vi "Pulse Generator.vi"() -> ()   [LabVIEW 2012]
uses:
  <vilib>/DAQmx/read.llb/DAQmx Read (Digital Bool 1Line 1Point).vi
  <vilib>/Utility/file.llb/Write To Spreadsheet File (DBL).vi
  <vilib>/DAQmx/create/channels.llb/DAQmx Create Channel (DI-Digital Input).vi
  <vilib>/DAQmx/miscellaneous.llb/DAQmx Fill In Error Info.vi
panel:
  in  "Tab Control":T1(tab)
  in  "MW width Min":dbl=5e-08
  in  "MW width step size":dbl=2e-09
  in  "MW width Max":dbl=5e-07
  in  "Tau step size":dbl
  in  "Tau max":dbl
  in  "Tau min":dbl
  in  "Rabi Frequency":dbl
  in  "Rabi Frequency":dbl
  in  "Tau max":dbl
  in  "Tau min":dbl
  in  "Tau step size":dbl
  in  "Tau":dbl
  in  "Rabi Frequency  2":dbl
  in  "Tau' max 2":dbl
  in  "Tau' min 2":dbl
  in  "Tau' step size 2":dbl
  in  "AOM Rest time":dbl
  in  "Signal delay":dbl
  in  "N Loop":i32=25000
  in  "APD signal width":dbl
  out "Run":bool
  out "size(s)":i32=225
  in  "file path (dialog if empty)":path=path "C:/Users/Ouyang Group/Documents/Data/12-5-13/Rabi pulse sequence 7"
  in  "AOM Pulse length":dbl=3e-07
  in  "Path to spinapi.dll":path=path "C:/SpinCore/SpinAPI/dll/spinapi64.dll"
  in  "stop":bool
  in  "start/restart":bool
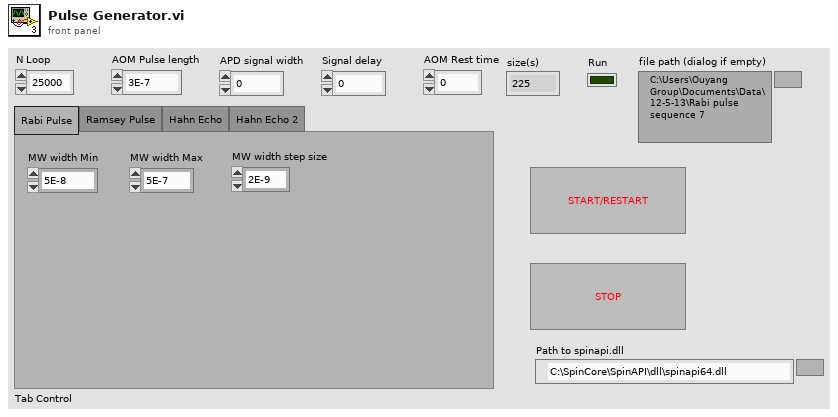
[diagram p1: front panel]
types:
  T1 = enum32{"Rabi Pulse", "Ramsey Pulse", "Hahn Echo", "Hahn Echo 2"}
  T2 = cluster{"Instruct Data":i32, "Op Code":i32, "Flags":bool[], "Comments":string, "Time (s)":dbl}[]
  T3 = cluster{"Instruct Data":i32, "Op Code":i32, "Flags":bool[], "Comments":string, "Time (s)":dbl}
  T4 = enum16{"Pulse Program", "Frequency Registers", "TX Phase Registers", "RX Phase Registers"}
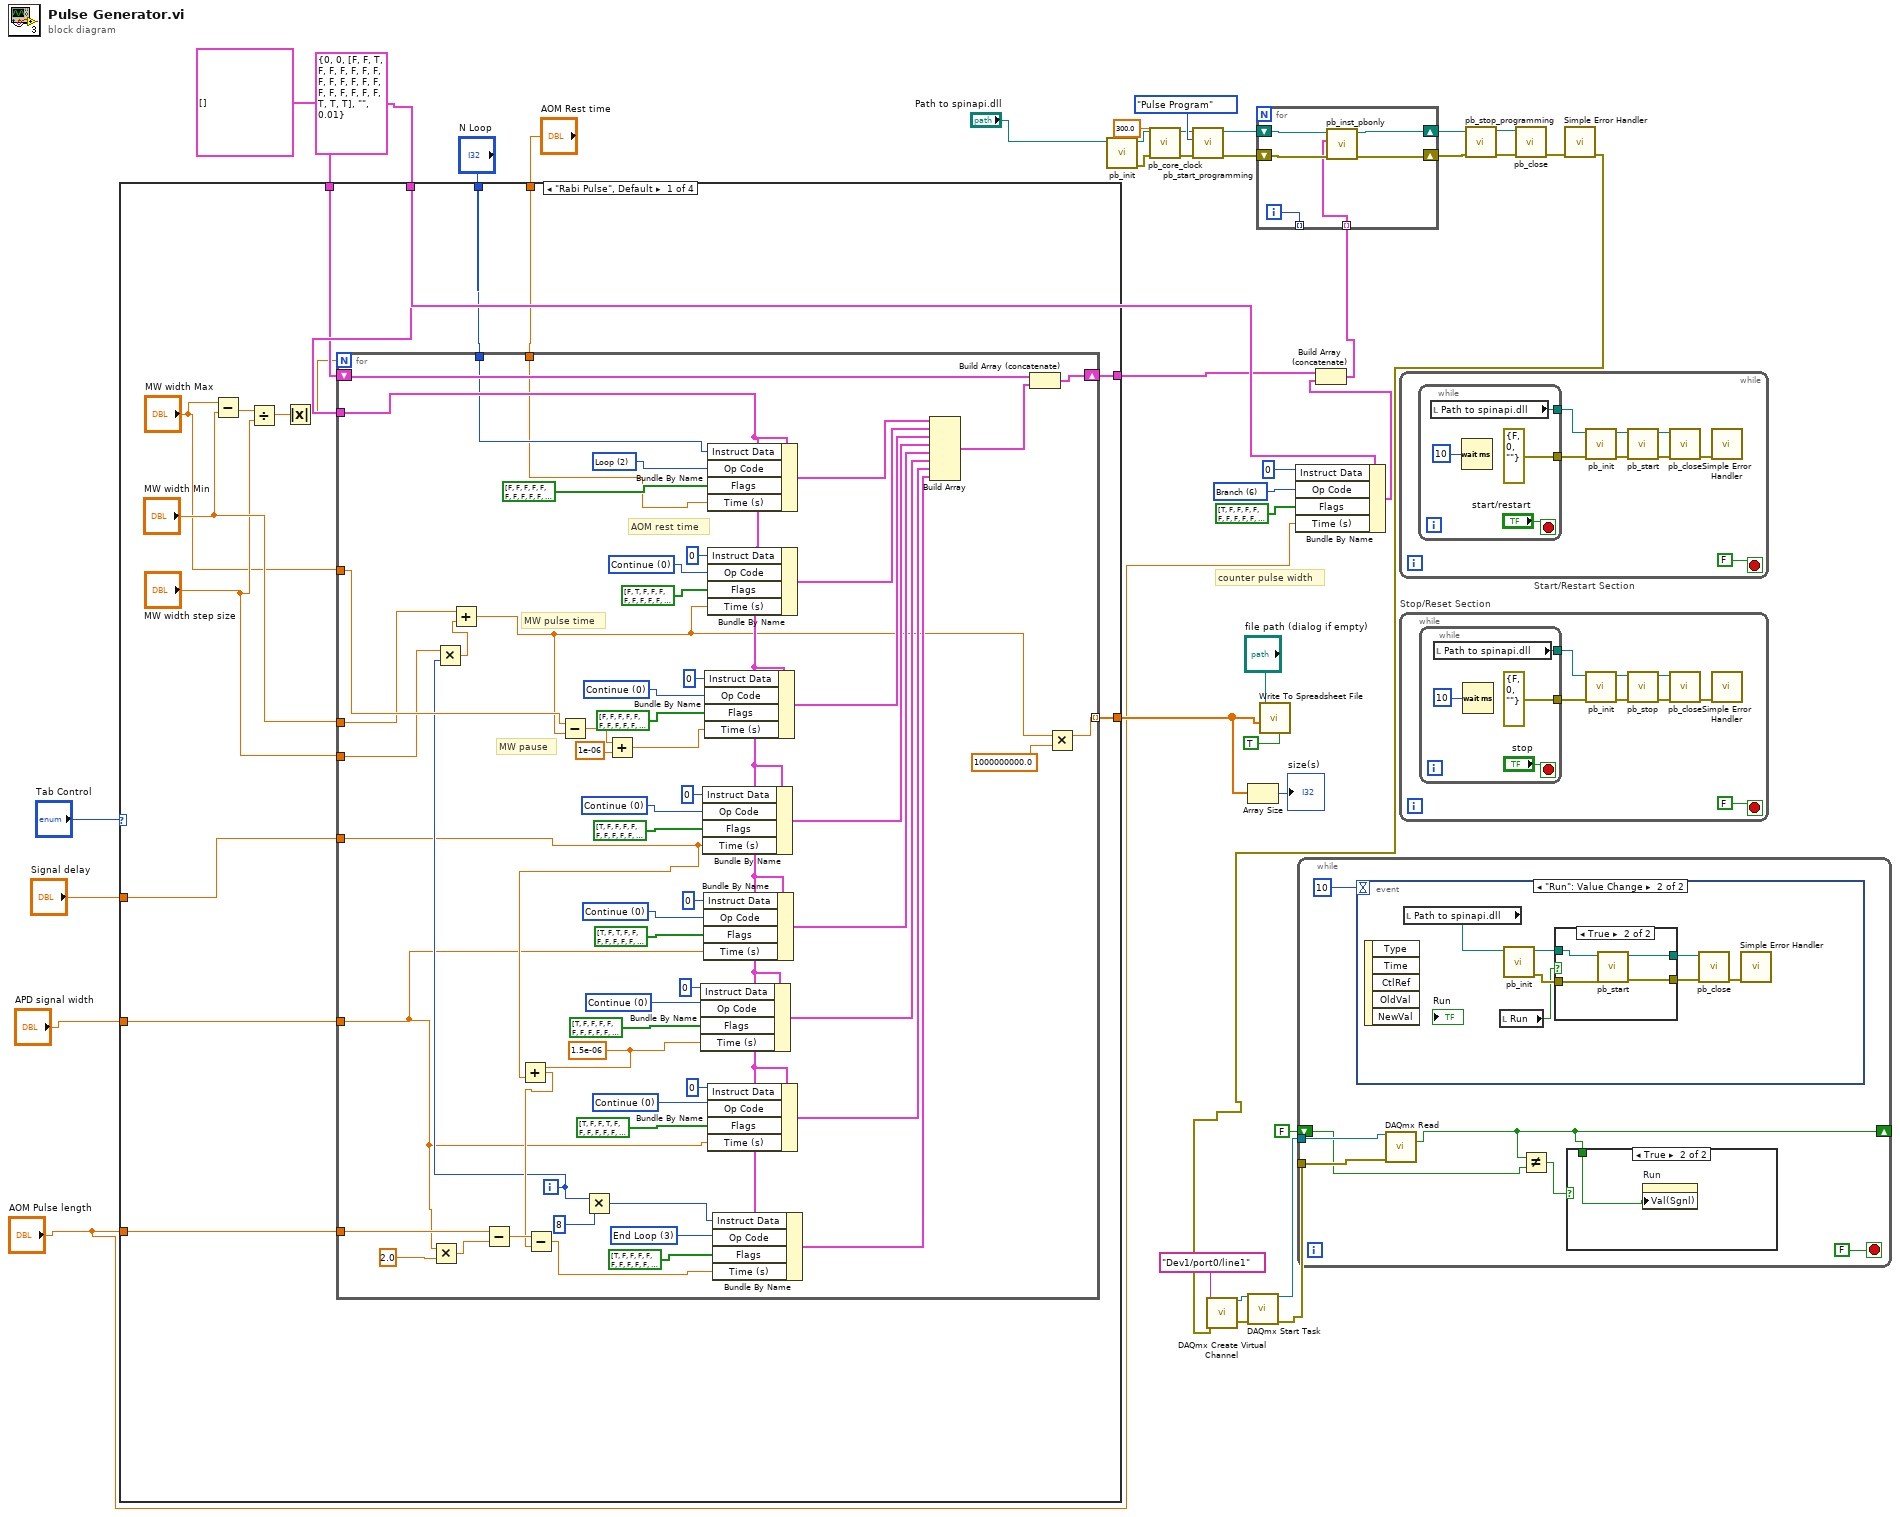
[diagram p0: block diagram]
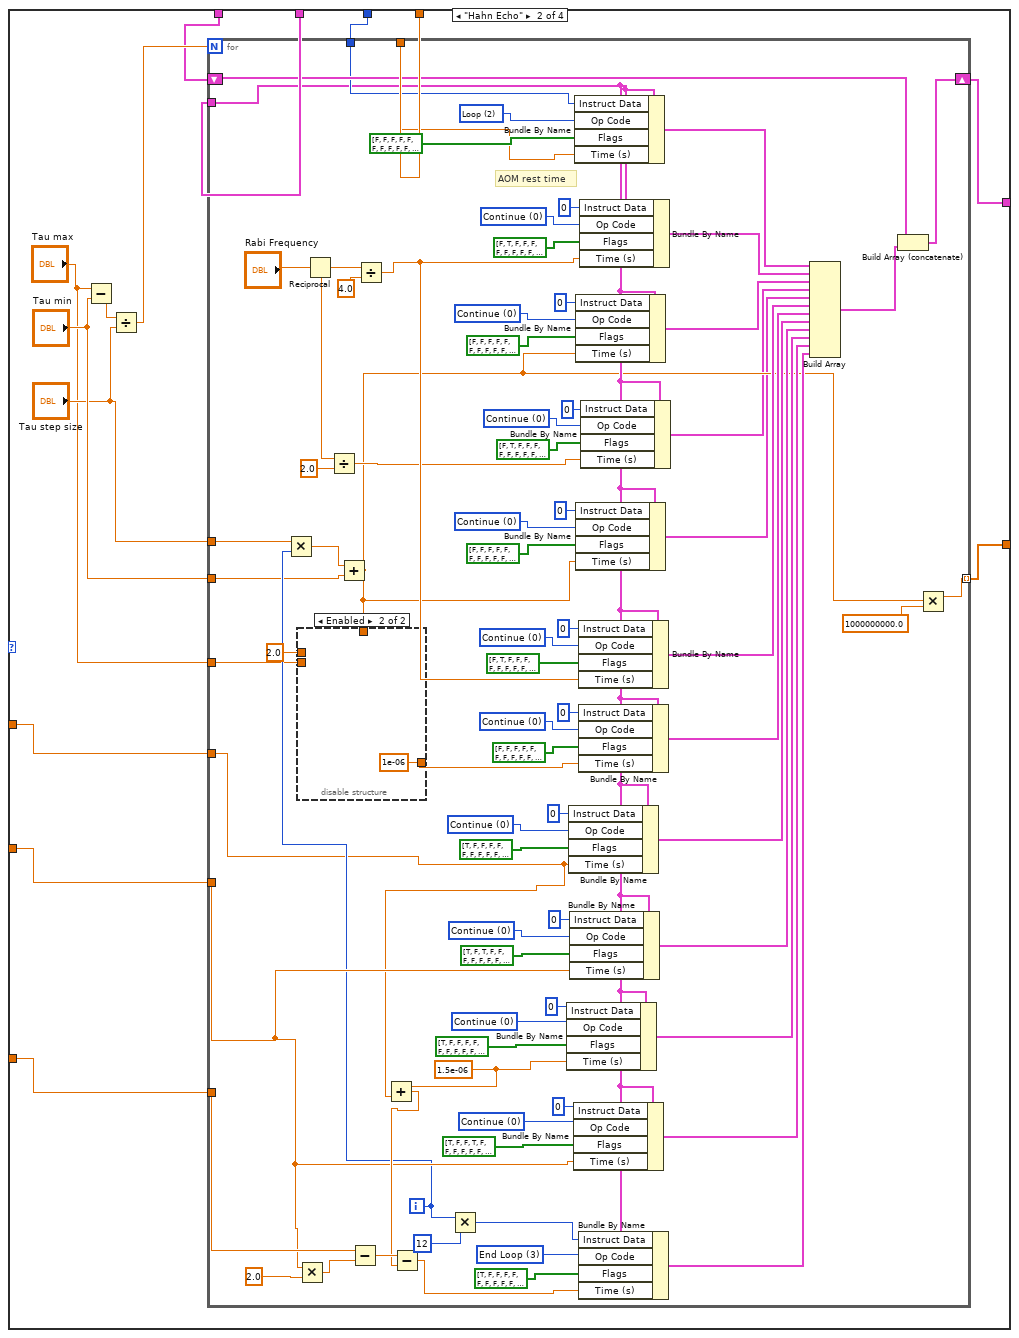
[diagram p2: hidden frame]
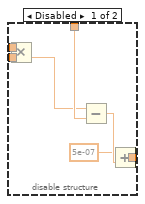
[diagram p3: hidden frame]
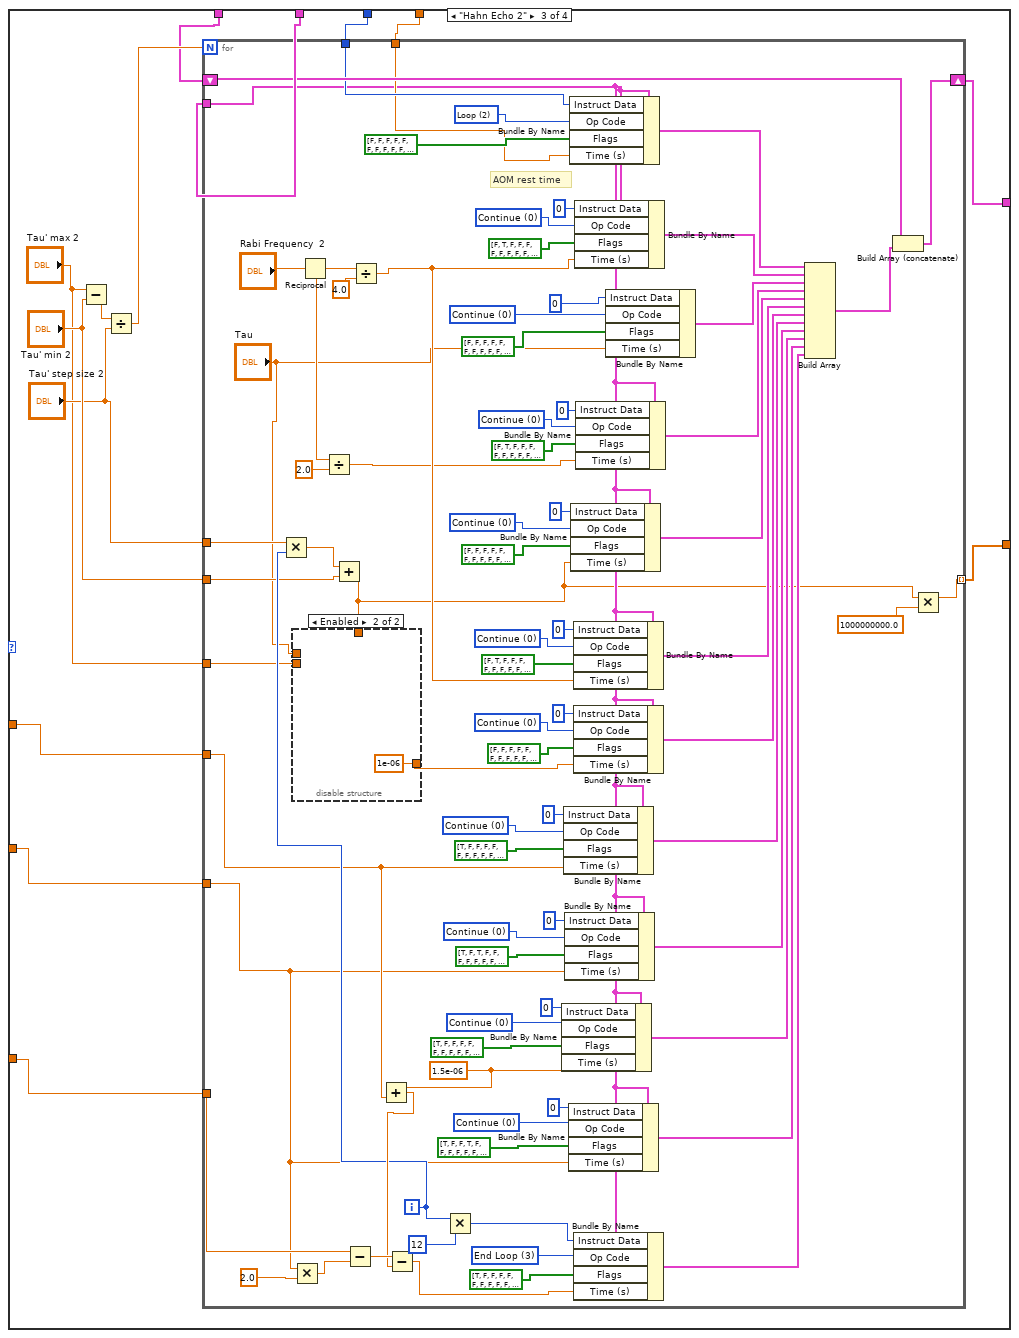
[diagram p4: hidden frame]
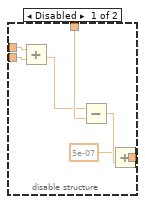
[diagram p5: hidden frame]
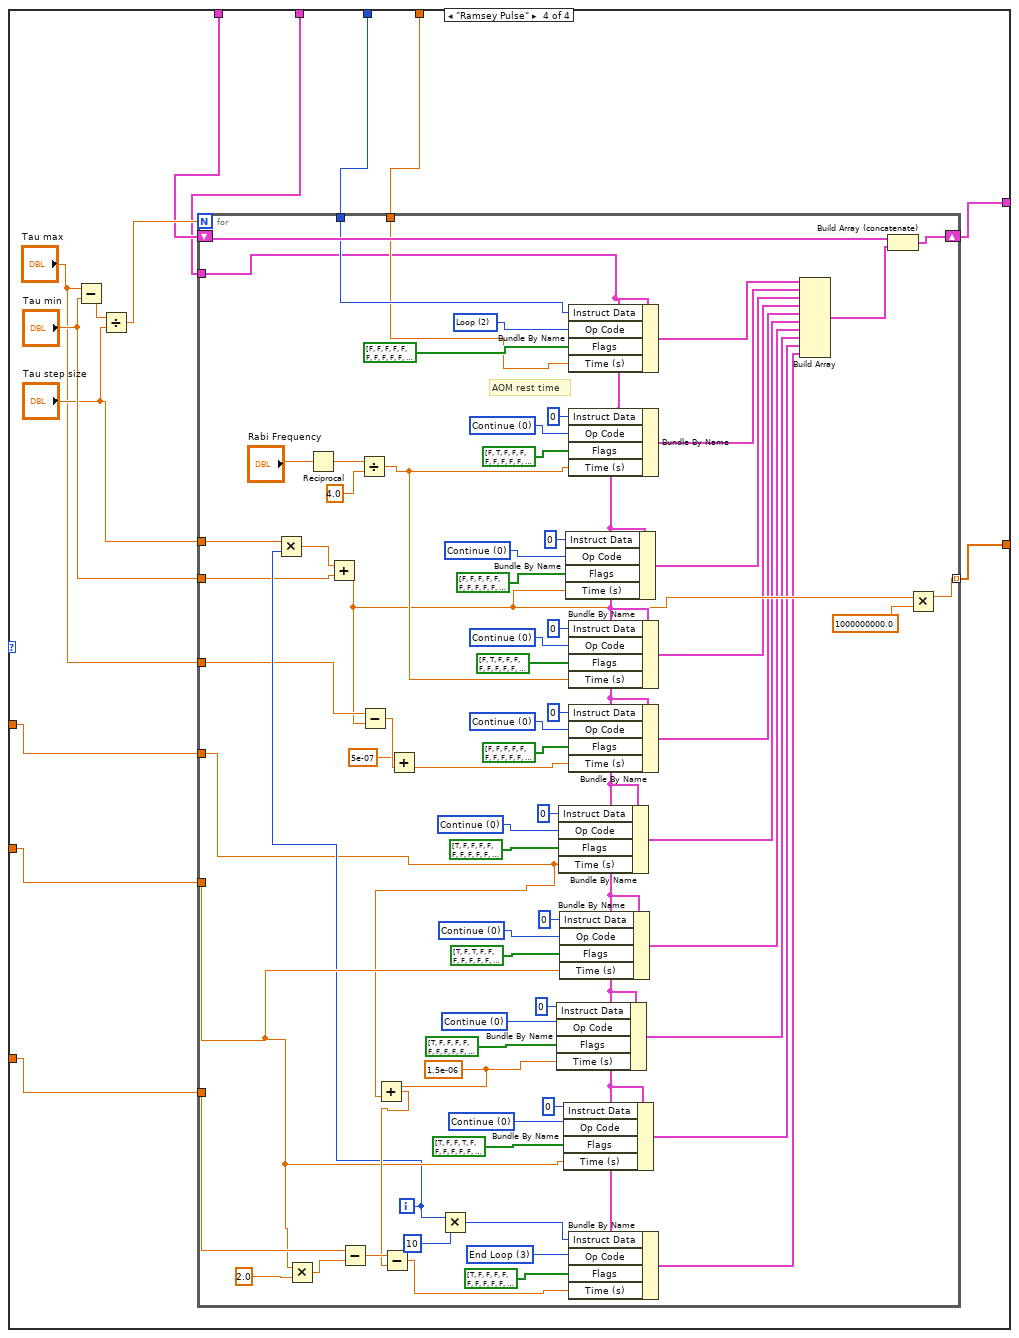
[diagram p6: hidden frame]
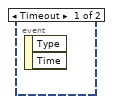
[diagram p7: hidden frame]
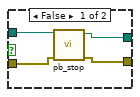
[diagram p8: hidden frame]
diagram:
  w13 = 6 items=["Continue", "Stop", "Loop", "End Loop", "JSR", "RTS", "Branch", "Long Delay", "Wait"] ("Op Code")
  w11 = T3 {"Instruct Data"=0, "Op Code"=0, "Flags"=[FALSE, FALSE, TRUE, FALSE, FALSE, FALSE, FALSE, FALSE, FALSE, FALSE, FALSE, FALSE, FALSE, FALSE, FALSE, FALSE, FALSE, FALSE, FALSE, FALSE, FALSE, TRUE, TRUE, TRUE], "Comments"="", "Time (s)"=0.01} ("PB Inst 2")
  # "counter pulse width"
  n1 = case shown="\"Rabi Pulse\", Default" "Tab Control" {
    tunnel: [w50 w115 w219 w328] -> w23
    tunnel: w11 -> [w48 w117 w222 w316]
    tunnel: [w47 w113 w220 w315] -> w9
    tunnel: T2 [] -> [w46 w118 w221 w317]
    tunnel: "N Loop" -> [w44 w116 w215 w327]
    tunnel: "AOM Rest time" -> [w43 w114 w214 w326]
    tunnel: "Signal delay" -> [w42 w121 w218 w323]
    tunnel: "AOM Pulse length" -> [w41 w119 w216 w325]
    tunnel: "APD signal width" -> [w40 w120 w217 w324]
    frame "Rabi Pulse", Default {
      n2 = Subtract(x="MW width Max", y="MW width Min") -> (x-y=w54:dbl)
      n3 = Divide(x=w54, y="MW width step size") -> (x/y=w53:dbl)
      n4 = Absolute Value(x=w53) -> (abs(x)=w45:dbl)
      n5 = for {
        N: w45 -> [_]
        tunnel: "MW width Min" -> [w61]
        tunnel: "MW width step size" -> [w62]
        tunnel: [w100] -> w50 mode=indexing
        tunnel: w48 -> [w81]
        shift-right: [w111] -> w47
        shift-left: w46 -> [w112]
        tunnel: "MW width Max" -> [w69]
        tunnel: w44 -> [w59]
        tunnel: w43 -> [w58]
        tunnel: w42 -> [w57]
        tunnel: w41 -> [w56]
        tunnel: w40 -> [w55]
        i -> [w63]
        w71 = 0 items=["Continue", "Stop", "Loop", "End Loop", "JSR", "RTS", "Branch", "Long Delay", "Wait"] ("Op Code")
        w74 = 2 items=["Continue", "Stop", "Loop", "End Loop", "JSR", "RTS", "Branch", "Long Delay", "Wait"] ("Op Code")
        w83 = 0 items=["Continue", "Stop", "Loop", "End Loop", "JSR", "RTS", "Branch", "Long Delay", "Wait"] ("Op Code")
        w86 = 1.5e-06 ("Time (s)")
        w90 = 0 items=["Continue", "Stop", "Loop", "End Loop", "JSR", "RTS", "Branch", "Long Delay", "Wait"] ("Op Code")
        w95 = 3 items=["Continue", "Stop", "Loop", "End Loop", "JSR", "RTS", "Branch", "Long Delay", "Wait"] ("Op Code")
        w98 = 0 items=["Continue", "Stop", "Loop", "End Loop", "JSR", "RTS", "Branch", "Long Delay", "Wait"] ("Op Code")
        w106 = 0 items=["Continue", "Stop", "Loop", "End Loop", "JSR", "RTS", "Branch", "Long Delay", "Wait"] ("Op Code")
        w109 = 0 items=["Continue", "Stop", "Loop", "End Loop", "JSR", "RTS", "Branch", "Long Delay", "Wait"] ("Op Code")
        # "MW pause"
        # "AOM rest time"
        # "MW pulse time"
        n6 = Multiply(x=w55, y=2.0) -> (x*y=w91:dbl)
        n7 = Multiply(x=w62, y=w63) -> (x*y=w64:dbl)
        n8 = Add(x=w61, y=w64) -> (x+y=w60:dbl)
        n9 = Subtract(x=w56, y=w91) -> (x-y=w87:dbl)
        n10 = Add(x=w86, y=w57) -> (x+y=w75:dbl)
        n11 = Subtract(x=w87, y=w75) -> (x-y=w85:dbl)
        n12 = Subtract(x=w69, y=w60) -> (x-y=w68:dbl)
        n13 = Multiply(x=w63, y=8) -> (x*y=w65:i32)
        n14 = Add(x=w68, y=1e-06) -> (x+y=w66:dbl)
        n15 = Bundle By Name(cluster=w81, "Instruct Data"=0, "Op Code"=w98, "Flags"=bool[] [TRUE, FALSE, FALSE, FALSE, FALSE, FALSE, FALSE, FALSE, FALSE, FALSE, FALSE, FALSE, FALSE, FALSE, FALSE, FALSE, FALSE, FALSE, FALSE, FALSE, FALSE, TRUE, TRUE, TRUE], "Time (s)"=w86) -> (w76:T3)
        n16 = Bundle By Name(cluster=w81, "Instruct Data"=0, "Op Code"=w83, "Flags"=bool[] [TRUE, FALSE, FALSE, FALSE, FALSE, FALSE, FALSE, FALSE, FALSE, FALSE, FALSE, FALSE, FALSE, FALSE, FALSE, FALSE, FALSE, FALSE, FALSE, FALSE, FALSE, TRUE, TRUE, TRUE], "Time (s)"=w57) -> (w79:T3)
        n17 = Bundle By Name(cluster=w81, "Instruct Data"=0, "Op Code"=w106, "Flags"=bool[] [TRUE, FALSE, TRUE, FALSE, FALSE, FALSE, FALSE, FALSE, FALSE, FALSE, FALSE, FALSE, FALSE, FALSE, FALSE, FALSE, FALSE, FALSE, FALSE, FALSE, FALSE, TRUE, TRUE, TRUE], "Time (s)"=w55) -> (w80:T3)
        n18 = Bundle By Name(cluster=w81, "Instruct Data"=0, "Op Code"=w109, "Flags"=bool[] [FALSE, FALSE, FALSE, FALSE, FALSE, FALSE, FALSE, FALSE, FALSE, FALSE, FALSE, FALSE, FALSE, FALSE, FALSE, FALSE, FALSE, FALSE, FALSE, FALSE, FALSE, TRUE, TRUE, TRUE], "Time (s)"=w66) -> (w103:T3)
        n19 = Bundle By Name(cluster=w81, "Instruct Data"=w59, "Op Code"=w74, "Flags"=bool[] [FALSE, FALSE, FALSE, FALSE, FALSE, FALSE, FALSE, FALSE, FALSE, FALSE, FALSE, FALSE, FALSE, FALSE, FALSE, FALSE, FALSE, FALSE, FALSE, FALSE, FALSE, TRUE, TRUE, TRUE], "Time (s)"=w58) -> (w105:T3)
        n20 = Bundle By Name(cluster=w81, "Instruct Data"=0, "Op Code"=w71, "Flags"=bool[] [FALSE, TRUE, FALSE, FALSE, FALSE, FALSE, FALSE, FALSE, FALSE, FALSE, FALSE, FALSE, FALSE, FALSE, FALSE, FALSE, FALSE, FALSE, FALSE, FALSE, FALSE, TRUE, TRUE, TRUE], "Time (s)"=w60) -> (w104:T3)
        n21 = Bundle By Name(cluster=w81, "Instruct Data"=0, "Op Code"=w90, "Flags"=bool[] [TRUE, FALSE, FALSE, TRUE, FALSE, FALSE, FALSE, FALSE, FALSE, FALSE, FALSE, FALSE, FALSE, FALSE, FALSE, FALSE, FALSE, FALSE, FALSE, FALSE, FALSE, TRUE, TRUE, TRUE], "Time (s)"=w55) -> (w77:T3)
        n22 = Bundle By Name(cluster=w81, "Instruct Data"=w65, "Op Code"=w95, "Flags"=bool[] [TRUE, FALSE, FALSE, FALSE, FALSE, FALSE, FALSE, FALSE, FALSE, FALSE, FALSE, FALSE, FALSE, FALSE, FALSE, FALSE, FALSE, FALSE, FALSE, FALSE, FALSE, TRUE, TRUE, TRUE], "Time (s)"=w85) -> (w78:T3)
        n23 = Build Array(w105, w104, w103, w79, w80, w76, w77, w78) -> (w101:T2)
        n24 = Build Array (concatenate)(w112, w101) -> (w111:T2)
        n25 = Multiply(x=w60, y=1000000000.0) -> (x*y=w100:dbl)
      }
    }
    frame "Hahn Echo" {
      n26 = Subtract(x="Tau max", y="Tau min") -> (x-y=w126:dbl)
      n27 = Divide(x=w126, y="Tau step size") -> (x/y=w125:dbl)
      n28 = for {
        N: w125 -> [_]
        tunnel: [w197] -> w115 mode=indexing
        tunnel: w117 -> [w134]
        shift-right: [w146] -> w113
        shift-left: w118 -> [w205]
        tunnel: w116 -> [w171]
        tunnel: w114 -> [w170]
        tunnel: w121 -> [w145]
        tunnel: w119 -> [w169]
        tunnel: w120 -> [w168]
        tunnel: "Tau min" -> [w165]
        tunnel: "Tau step size" -> [w167]
        tunnel: "Tau max" -> [w154]
        i -> [w166]
        w136 = 0 items=["Continue", "Stop", "Loop", "End Loop", "JSR", "RTS", "Branch", "Long Delay", "Wait"] ("Op Code")
        w142 = 0 items=["Continue", "Stop", "Loop", "End Loop", "JSR", "RTS", "Branch", "Long Delay", "Wait"] ("Op Code")
        w156 = 0 items=["Continue", "Stop", "Loop", "End Loop", "JSR", "RTS", "Branch", "Long Delay", "Wait"] ("Op Code")
        w160 = 0 items=["Continue", "Stop", "Loop", "End Loop", "JSR", "RTS", "Branch", "Long Delay", "Wait"] ("Op Code")
        w174 = 0 items=["Continue", "Stop", "Loop", "End Loop", "JSR", "RTS", "Branch", "Long Delay", "Wait"] ("Op Code")
        w177 = 2 items=["Continue", "Stop", "Loop", "End Loop", "JSR", "RTS", "Branch", "Long Delay", "Wait"] ("Op Code")
        w180 = 0 items=["Continue", "Stop", "Loop", "End Loop", "JSR", "RTS", "Branch", "Long Delay", "Wait"] ("Op Code")
        w183 = 1.5e-06 ("Time (s)")
        w187 = 0 items=["Continue", "Stop", "Loop", "End Loop", "JSR", "RTS", "Branch", "Long Delay", "Wait"] ("Op Code")
        w192 = 3 items=["Continue", "Stop", "Loop", "End Loop", "JSR", "RTS", "Branch", "Long Delay", "Wait"] ("Op Code")
        w195 = 0 items=["Continue", "Stop", "Loop", "End Loop", "JSR", "RTS", "Branch", "Long Delay", "Wait"] ("Op Code")
        w200 = 0 items=["Continue", "Stop", "Loop", "End Loop", "JSR", "RTS", "Branch", "Long Delay", "Wait"] ("Op Code")
        w203 = 0 items=["Continue", "Stop", "Loop", "End Loop", "JSR", "RTS", "Branch", "Long Delay", "Wait"] ("Op Code")
        # "AOM rest time"
        n29 = Multiply(x=w167, y=w166) -> (x*y=w164:dbl)
        n30 = Multiply(x=w168, y=2.0) -> (x*y=w188:dbl)
        n31 = Reciprocal(x="Rabi Frequency") -> (1/x=w140:dbl)
        n32 = Divide(x=w140, y=2.0) -> (x/y=w138:dbl)
        n33 = Add(x=w164, y=w165) -> (x+y=w133:dbl)
        n34 = disable-structure shown="Enabled" {
          disable-tunnel: w154 -> [w212 _]
          disable-tunnel: [w210 1e-06] -> w144
          disable-tunnel: w133 -> [w208 _]
          disable-tunnel: 2.0 ("x") -> [w206 _]
          frame Disabled {
            n35 = Multiply(x=w206, y=w212) -> (x*y=w207:dbl)
            n36 = Subtract(x=w207, y=w208) -> (x-y=w211:dbl)
            n37 = Add(x=5e-07, y=w211) -> (x+y=w210:dbl)
          }
          frame Enabled {
          }
        }
        n38 = Subtract(x=w169, y=w188) -> (x-y=w184:dbl)
        n39 = Divide(x=w140, y=4.0) -> (x/y=w158:dbl)
        n40 = Add(x=w183, y=w145) -> (x+y=w178:dbl)
        n41 = Subtract(x=w184, y=w178) -> (x-y=w182:dbl)
        n42 = Multiply(x=w166, y=12) -> (x*y=w172:i32)
        n43 = Bundle By Name(cluster=w134, "Instruct Data"=0, "Op Code"=w195, "Flags"=bool[] [TRUE, FALSE, FALSE, FALSE, FALSE, FALSE, FALSE, FALSE, FALSE, FALSE, FALSE, FALSE, FALSE, FALSE, FALSE, FALSE, FALSE, FALSE, FALSE, FALSE, FALSE, TRUE, TRUE, TRUE], "Time (s)"=w183) -> (w149:T3)
        n44 = Bundle By Name(cluster=w134, "Instruct Data"=0, "Op Code"=w180, "Flags"=bool[] [TRUE, FALSE, FALSE, FALSE, FALSE, FALSE, FALSE, FALSE, FALSE, FALSE, FALSE, FALSE, FALSE, FALSE, FALSE, FALSE, FALSE, FALSE, FALSE, FALSE, FALSE, TRUE, TRUE, TRUE], "Time (s)"=w145) -> (w151:T3)
        n45 = Bundle By Name(cluster=w134, "Instruct Data"=0, "Op Code"=w200, "Flags"=bool[] [TRUE, FALSE, TRUE, FALSE, FALSE, FALSE, FALSE, FALSE, FALSE, FALSE, FALSE, FALSE, FALSE, FALSE, FALSE, FALSE, FALSE, FALSE, FALSE, FALSE, FALSE, TRUE, TRUE, TRUE], "Time (s)"=w168) -> (w150:T3)
        n46 = Bundle By Name(cluster=w134, "Instruct Data"=0, "Op Code"=w187, "Flags"=bool[] [TRUE, FALSE, FALSE, TRUE, FALSE, FALSE, FALSE, FALSE, FALSE, FALSE, FALSE, FALSE, FALSE, FALSE, FALSE, FALSE, FALSE, FALSE, FALSE, FALSE, FALSE, TRUE, TRUE, TRUE], "Time (s)"=w168) -> (w148:T3)
        n47 = Bundle By Name(cluster=w134, "Instruct Data"=w171, "Op Code"=w177, "Flags"=bool[] [FALSE, FALSE, FALSE, FALSE, FALSE, FALSE, FALSE, FALSE, FALSE, FALSE, FALSE, FALSE, FALSE, FALSE, FALSE, FALSE, FALSE, FALSE, FALSE, FALSE, FALSE, TRUE, TRUE, TRUE], "Time (s)"=w170) -> (w127:T3)
        n48 = Bundle By Name(cluster=w134, "Instruct Data"=0, "Op Code"=w203, "Flags"=bool[] [FALSE, FALSE, FALSE, FALSE, FALSE, FALSE, FALSE, FALSE, FALSE, FALSE, FALSE, FALSE, FALSE, FALSE, FALSE, FALSE, FALSE, FALSE, FALSE, FALSE, FALSE, TRUE, TRUE, TRUE], "Time (s)"=w133) -> (w129:T3)
        n49 = Bundle By Name(cluster=w134, "Instruct Data"=0, "Op Code"=w136, "Flags"=bool[] [FALSE, FALSE, FALSE, FALSE, FALSE, FALSE, FALSE, FALSE, FALSE, FALSE, FALSE, FALSE, FALSE, FALSE, FALSE, FALSE, FALSE, FALSE, FALSE, FALSE, FALSE, TRUE, TRUE, TRUE], "Time (s)"=w133) -> (w131:T3)
        n50 = Bundle By Name(cluster=w134, "Instruct Data"=0, "Op Code"=w160, "Flags"=bool[] [FALSE, TRUE, FALSE, FALSE, FALSE, FALSE, FALSE, FALSE, FALSE, FALSE, FALSE, FALSE, FALSE, FALSE, FALSE, FALSE, FALSE, FALSE, FALSE, FALSE, FALSE, TRUE, TRUE, TRUE], "Time (s)"=w158) -> (w153:T3)
        n51 = Bundle By Name(cluster=w134, "Instruct Data"=0, "Op Code"=w156, "Flags"=bool[] [FALSE, FALSE, FALSE, FALSE, FALSE, FALSE, FALSE, FALSE, FALSE, FALSE, FALSE, FALSE, FALSE, FALSE, FALSE, FALSE, FALSE, FALSE, FALSE, FALSE, FALSE, TRUE, TRUE, TRUE], "Time (s)"=w144) -> (w152:T3)
        n52 = Bundle By Name(cluster=w134, "Instruct Data"=w172, "Op Code"=w192, "Flags"=bool[] [TRUE, FALSE, FALSE, FALSE, FALSE, FALSE, FALSE, FALSE, FALSE, FALSE, FALSE, FALSE, FALSE, FALSE, FALSE, FALSE, FALSE, FALSE, FALSE, FALSE, FALSE, TRUE, TRUE, TRUE], "Time (s)"=w182) -> (w147:T3)
        n53 = Bundle By Name(cluster=w134, "Instruct Data"=0, "Op Code"=w174, "Flags"=bool[] [FALSE, TRUE, FALSE, FALSE, FALSE, FALSE, FALSE, FALSE, FALSE, FALSE, FALSE, FALSE, FALSE, FALSE, FALSE, FALSE, FALSE, FALSE, FALSE, FALSE, FALSE, TRUE, TRUE, TRUE], "Time (s)"=w158) -> (w128:T3)
        n54 = Bundle By Name(cluster=w134, "Instruct Data"=0, "Op Code"=w142, "Flags"=bool[] [FALSE, TRUE, FALSE, FALSE, FALSE, FALSE, FALSE, FALSE, FALSE, FALSE, FALSE, FALSE, FALSE, FALSE, FALSE, FALSE, FALSE, FALSE, FALSE, FALSE, FALSE, TRUE, TRUE, TRUE], "Time (s)"=w138) -> (w130:T3)
        n55 = Build Array(w127, w128, w129, w130, w131, w153, w152, w151, w150, w149, w148, w147) -> (w198:T2)
        n56 = Build Array (concatenate)(w205, w198) -> (w146:T2)
        n57 = Multiply(x=w133, y=1000000000.0) -> (x*y=w197:dbl)
      }
    }
    frame "Hahn Echo 2" {
      n58 = Subtract(x="Tau' max 2", y="Tau' min 2") -> (x-y=w227:dbl)
      n59 = Divide(x=w227, y="Tau' step size 2") -> (x/y=w226:dbl)
      n60 = for {
        N: w226 -> [_]
        tunnel: [w298] -> w219 mode=indexing
        tunnel: w222 -> [w236]
        shift-right: [w248] -> w220
        shift-left: w221 -> [w306]
        tunnel: w215 -> [w272]
        tunnel: w214 -> [w271]
        tunnel: w218 -> [w247]
        tunnel: w216 -> [w270]
        tunnel: w217 -> [w228]
        tunnel: "Tau' min 2" -> [w267]
        tunnel: "Tau' step size 2" -> [w269]
        tunnel: "Tau' max 2" -> [w256]
        i -> [w268]
        w238 = 0 items=["Continue", "Stop", "Loop", "End Loop", "JSR", "RTS", "Branch", "Long Delay", "Wait"] ("Op Code")
        w244 = 0 items=["Continue", "Stop", "Loop", "End Loop", "JSR", "RTS", "Branch", "Long Delay", "Wait"] ("Op Code")
        w258 = 0 items=["Continue", "Stop", "Loop", "End Loop", "JSR", "RTS", "Branch", "Long Delay", "Wait"] ("Op Code")
        w262 = 0 items=["Continue", "Stop", "Loop", "End Loop", "JSR", "RTS", "Branch", "Long Delay", "Wait"] ("Op Code")
        w275 = 0 items=["Continue", "Stop", "Loop", "End Loop", "JSR", "RTS", "Branch", "Long Delay", "Wait"] ("Op Code")
        w278 = 2 items=["Continue", "Stop", "Loop", "End Loop", "JSR", "RTS", "Branch", "Long Delay", "Wait"] ("Op Code")
        w281 = 0 items=["Continue", "Stop", "Loop", "End Loop", "JSR", "RTS", "Branch", "Long Delay", "Wait"] ("Op Code")
        w284 = 1.5e-06 ("Time (s)")
        w288 = 0 items=["Continue", "Stop", "Loop", "End Loop", "JSR", "RTS", "Branch", "Long Delay", "Wait"] ("Op Code")
        w293 = 3 items=["Continue", "Stop", "Loop", "End Loop", "JSR", "RTS", "Branch", "Long Delay", "Wait"] ("Op Code")
        w296 = 0 items=["Continue", "Stop", "Loop", "End Loop", "JSR", "RTS", "Branch", "Long Delay", "Wait"] ("Op Code")
        w301 = 0 items=["Continue", "Stop", "Loop", "End Loop", "JSR", "RTS", "Branch", "Long Delay", "Wait"] ("Op Code")
        w304 = 0 items=["Continue", "Stop", "Loop", "End Loop", "JSR", "RTS", "Branch", "Long Delay", "Wait"] ("Op Code")
        # "AOM rest time"
        n61 = Multiply(x=w269, y=w268) -> (x*y=w266:dbl)
        n62 = Multiply(x=w228, y=2.0) -> (x*y=w289:dbl)
        n63 = Reciprocal(x="Rabi Frequency  2") -> (1/x=w242:dbl)
        n64 = Divide(x=w242, y=2.0) -> (x/y=w240:dbl)
        n65 = Add(x=w266, y=w267) -> (x+y=w230:dbl)
        n66 = disable-structure shown="Enabled" {
          disable-tunnel: w256 -> [w313 _]
          disable-tunnel: [w311 1e-06] -> w246
          disable-tunnel: w230 -> [w309 _]
          disable-tunnel: "Tau" -> [w307 _]
          frame Disabled {
            n67 = Add(x=w307, y=w313) -> (x+y=w308:dbl)
            n68 = Subtract(x=w308, y=w309) -> (x-y=w312:dbl)
            n69 = Add(x=5e-07, y=w312) -> (x+y=w311:dbl)
          }
          frame Enabled {
          }
        }
        n70 = Subtract(x=w270, y=w289) -> (x-y=w285:dbl)
        n71 = Divide(x=w242, y=4.0) -> (x/y=w260:dbl)
        n72 = Add(x=w284, y=w247) -> (x+y=w279:dbl)
        n73 = Subtract(x=w285, y=w279) -> (x-y=w283:dbl)
        n74 = Multiply(x=w268, y=12) -> (x*y=w273:i32)
        n75 = Bundle By Name(cluster=w236, "Instruct Data"=0, "Op Code"=w296, "Flags"=bool[] [TRUE, FALSE, FALSE, FALSE, FALSE, FALSE, FALSE, FALSE, FALSE, FALSE, FALSE, FALSE, FALSE, FALSE, FALSE, FALSE, FALSE, FALSE, FALSE, FALSE, FALSE, TRUE, TRUE, TRUE], "Time (s)"=w284) -> (w251:T3)
        n76 = Bundle By Name(cluster=w236, "Instruct Data"=0, "Op Code"=w281, "Flags"=bool[] [TRUE, FALSE, FALSE, FALSE, FALSE, FALSE, FALSE, FALSE, FALSE, FALSE, FALSE, FALSE, FALSE, FALSE, FALSE, FALSE, FALSE, FALSE, FALSE, FALSE, FALSE, TRUE, TRUE, TRUE], "Time (s)"=w247) -> (w253:T3)
        n77 = Bundle By Name(cluster=w236, "Instruct Data"=0, "Op Code"=w301, "Flags"=bool[] [TRUE, FALSE, TRUE, FALSE, FALSE, FALSE, FALSE, FALSE, FALSE, FALSE, FALSE, FALSE, FALSE, FALSE, FALSE, FALSE, FALSE, FALSE, FALSE, FALSE, FALSE, TRUE, TRUE, TRUE], "Time (s)"=w228) -> (w252:T3)
        n78 = Bundle By Name(cluster=w236, "Instruct Data"=0, "Op Code"=w288, "Flags"=bool[] [TRUE, FALSE, FALSE, TRUE, FALSE, FALSE, FALSE, FALSE, FALSE, FALSE, FALSE, FALSE, FALSE, FALSE, FALSE, FALSE, FALSE, FALSE, FALSE, FALSE, FALSE, TRUE, TRUE, TRUE], "Time (s)"=w228) -> (w250:T3)
        n79 = Bundle By Name(cluster=w236, "Instruct Data"=w272, "Op Code"=w278, "Flags"=bool[] [FALSE, FALSE, FALSE, FALSE, FALSE, FALSE, FALSE, FALSE, FALSE, FALSE, FALSE, FALSE, FALSE, FALSE, FALSE, FALSE, FALSE, FALSE, FALSE, FALSE, FALSE, TRUE, TRUE, TRUE], "Time (s)"=w271) -> (w231:T3)
        n80 = Bundle By Name(cluster=w236, "Instruct Data"=0, "Op Code"=w238, "Flags"=bool[] [FALSE, FALSE, FALSE, FALSE, FALSE, FALSE, FALSE, FALSE, FALSE, FALSE, FALSE, FALSE, FALSE, FALSE, FALSE, FALSE, FALSE, FALSE, FALSE, FALSE, FALSE, TRUE, TRUE, TRUE], "Time (s)"=w230) -> (w235:T3)
        n81 = Bundle By Name(cluster=w236, "Instruct Data"=0, "Op Code"=w262, "Flags"=bool[] [FALSE, TRUE, FALSE, FALSE, FALSE, FALSE, FALSE, FALSE, FALSE, FALSE, FALSE, FALSE, FALSE, FALSE, FALSE, FALSE, FALSE, FALSE, FALSE, FALSE, FALSE, TRUE, TRUE, TRUE], "Time (s)"=w260) -> (w255:T3)
        n82 = Bundle By Name(cluster=w236, "Instruct Data"=0, "Op Code"=w258, "Flags"=bool[] [FALSE, FALSE, FALSE, FALSE, FALSE, FALSE, FALSE, FALSE, FALSE, FALSE, FALSE, FALSE, FALSE, FALSE, FALSE, FALSE, FALSE, FALSE, FALSE, FALSE, FALSE, TRUE, TRUE, TRUE], "Time (s)"=w246) -> (w254:T3)
        n83 = Bundle By Name(cluster=w236, "Instruct Data"=w273, "Op Code"=w293, "Flags"=bool[] [TRUE, FALSE, FALSE, FALSE, FALSE, FALSE, FALSE, FALSE, FALSE, FALSE, FALSE, FALSE, FALSE, FALSE, FALSE, FALSE, FALSE, FALSE, FALSE, FALSE, FALSE, TRUE, TRUE, TRUE], "Time (s)"=w283) -> (w249:T3)
        n84 = Bundle By Name(cluster=w236, "Instruct Data"=0, "Op Code"=w275, "Flags"=bool[] [FALSE, TRUE, FALSE, FALSE, FALSE, FALSE, FALSE, FALSE, FALSE, FALSE, FALSE, FALSE, FALSE, FALSE, FALSE, FALSE, FALSE, FALSE, FALSE, FALSE, FALSE, TRUE, TRUE, TRUE], "Time (s)"=w260) -> (w232:T3)
        n85 = Bundle By Name(cluster=w236, "Instruct Data"=0, "Op Code"=w244, "Flags"=bool[] [FALSE, TRUE, FALSE, FALSE, FALSE, FALSE, FALSE, FALSE, FALSE, FALSE, FALSE, FALSE, FALSE, FALSE, FALSE, FALSE, FALSE, FALSE, FALSE, FALSE, FALSE, TRUE, TRUE, TRUE], "Time (s)"=w240) -> (w234:T3)
        n86 = Bundle By Name(cluster=w236, "Instruct Data"=0, "Op Code"=w304, "Flags"=bool[] [FALSE, FALSE, FALSE, FALSE, FALSE, FALSE, FALSE, FALSE, FALSE, FALSE, FALSE, FALSE, FALSE, FALSE, FALSE, FALSE, FALSE, FALSE, FALSE, FALSE, FALSE, TRUE, TRUE, TRUE], "Time (s)"="Tau") -> (w233:T3)
        n87 = Build Array(w231, w232, w233, w234, w235, w255, w254, w253, w252, w251, w250, w249) -> (w299:T2)
        n88 = Build Array (concatenate)(w306, w299) -> (w248:T2)
        n89 = Multiply(x=w230, y=1000000000.0) -> (x*y=w298:dbl)
      }
    }
    frame "Ramsey Pulse" {
      n90 = Subtract(x="Tau max", y="Tau min") -> (x-y=w322:dbl)
      n91 = Divide(x=w322, y="Tau step size") -> (x/y=w321:dbl)
      n92 = for {
        N: w321 -> [_]
        tunnel: [w387] -> w328 mode=indexing
        tunnel: w316 -> [w343]
        shift-right: [w332] -> w315
        shift-left: w317 -> [w398]
        tunnel: w327 -> [w361]
        tunnel: w326 -> [w360]
        tunnel: w323 -> [w331]
        tunnel: w325 -> [w359]
        tunnel: w324 -> [w358]
        tunnel: "Tau min" -> [w355]
        tunnel: "Tau step size" -> [w357]
        tunnel: "Tau max" -> [w342]
        i -> [w356]
        w345 = 0 items=["Continue", "Stop", "Loop", "End Loop", "JSR", "RTS", "Branch", "Long Delay", "Wait"] ("Op Code")
        w349 = 0 items=["Continue", "Stop", "Loop", "End Loop", "JSR", "RTS", "Branch", "Long Delay", "Wait"] ("Op Code")
        w364 = 0 items=["Continue", "Stop", "Loop", "End Loop", "JSR", "RTS", "Branch", "Long Delay", "Wait"] ("Op Code")
        w367 = 2 items=["Continue", "Stop", "Loop", "End Loop", "JSR", "RTS", "Branch", "Long Delay", "Wait"] ("Op Code")
        w370 = 0 items=["Continue", "Stop", "Loop", "End Loop", "JSR", "RTS", "Branch", "Long Delay", "Wait"] ("Op Code")
        w373 = 1.5e-06 ("Time (s)")
        w377 = 0 items=["Continue", "Stop", "Loop", "End Loop", "JSR", "RTS", "Branch", "Long Delay", "Wait"] ("Op Code")
        w382 = 3 items=["Continue", "Stop", "Loop", "End Loop", "JSR", "RTS", "Branch", "Long Delay", "Wait"] ("Op Code")
        w385 = 0 items=["Continue", "Stop", "Loop", "End Loop", "JSR", "RTS", "Branch", "Long Delay", "Wait"] ("Op Code")
        w393 = 0 items=["Continue", "Stop", "Loop", "End Loop", "JSR", "RTS", "Branch", "Long Delay", "Wait"] ("Op Code")
        w396 = 0 items=["Continue", "Stop", "Loop", "End Loop", "JSR", "RTS", "Branch", "Long Delay", "Wait"] ("Op Code")
        # "AOM rest time"
        n93 = Multiply(x=w357, y=w356) -> (x*y=w354:dbl)
        n94 = Multiply(x=w358, y=2.0) -> (x*y=w378:dbl)
        n95 = Reciprocal(x="Rabi Frequency") -> (1/x=w352:dbl)
        n96 = Add(x=w354, y=w355) -> (x+y=w341:dbl)
        n97 = Subtract(x=w359, y=w378) -> (x-y=w374:dbl)
        n98 = Divide(x=w352, y=4.0) -> (x/y=w347:dbl)
        n99 = Subtract(x=w342, y=w341) -> (x-y=w340:dbl)
        n100 = Add(x=w373, y=w331) -> (x+y=w368:dbl)
        n101 = Subtract(x=w374, y=w368) -> (x-y=w372:dbl)
        n102 = Add(x=5e-07, y=w340) -> (x+y=w330:dbl)
        n103 = Multiply(x=w356, y=10) -> (x*y=w362:i32)
        n104 = Bundle By Name(cluster=w343, "Instruct Data"=0, "Op Code"=w385, "Flags"=bool[] [TRUE, FALSE, FALSE, FALSE, FALSE, FALSE, FALSE, FALSE, FALSE, FALSE, FALSE, FALSE, FALSE, FALSE, FALSE, FALSE, FALSE, FALSE, FALSE, FALSE, FALSE, TRUE, TRUE, TRUE], "Time (s)"=w373) -> (w335:T3)
        n105 = Bundle By Name(cluster=w343, "Instruct Data"=0, "Op Code"=w370, "Flags"=bool[] [TRUE, FALSE, FALSE, FALSE, FALSE, FALSE, FALSE, FALSE, FALSE, FALSE, FALSE, FALSE, FALSE, FALSE, FALSE, FALSE, FALSE, FALSE, FALSE, FALSE, FALSE, TRUE, TRUE, TRUE], "Time (s)"=w331) -> (w337:T3)
        n106 = Bundle By Name(cluster=w343, "Instruct Data"=0, "Op Code"=w393, "Flags"=bool[] [TRUE, FALSE, TRUE, FALSE, FALSE, FALSE, FALSE, FALSE, FALSE, FALSE, FALSE, FALSE, FALSE, FALSE, FALSE, FALSE, FALSE, FALSE, FALSE, FALSE, FALSE, TRUE, TRUE, TRUE], "Time (s)"=w358) -> (w336:T3)
        n107 = Bundle By Name(cluster=w343, "Instruct Data"=0, "Op Code"=w377, "Flags"=bool[] [TRUE, FALSE, FALSE, TRUE, FALSE, FALSE, FALSE, FALSE, FALSE, FALSE, FALSE, FALSE, FALSE, FALSE, FALSE, FALSE, FALSE, FALSE, FALSE, FALSE, FALSE, TRUE, TRUE, TRUE], "Time (s)"=w358) -> (w334:T3)
        n108 = Bundle By Name(cluster=w343, "Instruct Data"=0, "Op Code"=w396, "Flags"=bool[] [FALSE, FALSE, FALSE, FALSE, FALSE, FALSE, FALSE, FALSE, FALSE, FALSE, FALSE, FALSE, FALSE, FALSE, FALSE, FALSE, FALSE, FALSE, FALSE, FALSE, FALSE, TRUE, TRUE, TRUE], "Time (s)"=w341) -> (w390:T3)
        n109 = Bundle By Name(cluster=w343, "Instruct Data"=w361, "Op Code"=w367, "Flags"=bool[] [FALSE, FALSE, FALSE, FALSE, FALSE, FALSE, FALSE, FALSE, FALSE, FALSE, FALSE, FALSE, FALSE, FALSE, FALSE, FALSE, FALSE, FALSE, FALSE, FALSE, FALSE, TRUE, TRUE, TRUE], "Time (s)"=w360) -> (w392:T3)
        n110 = Bundle By Name(cluster=w343, "Instruct Data"=0, "Op Code"=w364, "Flags"=bool[] [FALSE, TRUE, FALSE, FALSE, FALSE, FALSE, FALSE, FALSE, FALSE, FALSE, FALSE, FALSE, FALSE, FALSE, FALSE, FALSE, FALSE, FALSE, FALSE, FALSE, FALSE, TRUE, TRUE, TRUE], "Time (s)"=w347) -> (w391:T3)
        n111 = Bundle By Name(cluster=w343, "Instruct Data"=0, "Op Code"=w349, "Flags"=bool[] [FALSE, TRUE, FALSE, FALSE, FALSE, FALSE, FALSE, FALSE, FALSE, FALSE, FALSE, FALSE, FALSE, FALSE, FALSE, FALSE, FALSE, FALSE, FALSE, FALSE, FALSE, TRUE, TRUE, TRUE], "Time (s)"=w347) -> (w339:T3)
        n112 = Bundle By Name(cluster=w343, "Instruct Data"=0, "Op Code"=w345, "Flags"=bool[] [FALSE, FALSE, FALSE, FALSE, FALSE, FALSE, FALSE, FALSE, FALSE, FALSE, FALSE, FALSE, FALSE, FALSE, FALSE, FALSE, FALSE, FALSE, FALSE, FALSE, FALSE, TRUE, TRUE, TRUE], "Time (s)"=w330) -> (w338:T3)
        n113 = Bundle By Name(cluster=w343, "Instruct Data"=w362, "Op Code"=w382, "Flags"=bool[] [TRUE, FALSE, FALSE, FALSE, FALSE, FALSE, FALSE, FALSE, FALSE, FALSE, FALSE, FALSE, FALSE, FALSE, FALSE, FALSE, FALSE, FALSE, FALSE, FALSE, FALSE, TRUE, TRUE, TRUE], "Time (s)"=w372) -> (w333:T3)
        n114 = Build Array(w392, w391, w390, w339, w338, w337, w336, w335, w334, w333) -> (w388:T2)
        n115 = Build Array (concatenate)(w398, w388) -> (w332:T2)
        n116 = Multiply(x=w341, y=1000000000.0) -> (x*y=w387:dbl)
      }
    }
  }
  n117 = call "pb_init.vi"("path in"="Path to spinapi.dll") -> ("error out"=w34:errorcluster, "path out"=w36:path)  [unwired: 3 in, 6 out]
  n118 = call "pb_core_clock.vi"("error in (no error)"=w34, "clock_freq (MHz)"=300.0, "path in"=w36) -> ("error out"=w33:errorcluster, "path out"=w35:path)  [unwired: 7 in]
  n119 = call "pb_start_programming.vi"("error in (no error)"=w33, "Device"=T4."Pulse Program", "path in"=w35) -> ("error out"=w30:errorcluster, "path out"=w31:path)  [unwired: 1 in, 6 out]
  n120 = Array Size(array=w23) -> (size(s)=→"size(s)":i32)
  n121 = call-poly <vilib>:"Write To Spreadsheet File.vi"("transpose? (no:F)"=TRUE, "1D data"=w23, "file path (dialog if empty)"="file path (dialog if empty)") -> ()  [unwired: 5 in, 1 out]
  n122 = Bundle By Name(cluster=w11, "Instruct Data"=0, "Op Code"=w13, "Flags"=bool[] [TRUE, FALSE, FALSE, FALSE, FALSE, FALSE, FALSE, FALSE, FALSE, FALSE, FALSE, FALSE, FALSE, FALSE, FALSE, FALSE, FALSE, FALSE, FALSE, FALSE, FALSE, TRUE, TRUE, TRUE], "Time (s)"="AOM Pulse length") -> (w10:T3)
  n123 = Build Array (concatenate)(w9, w10) -> (w8:T2)
  n124 = for {
    shift-right: [w402] -> w29
    shift-left: w31 -> [w404]
    shift-right: [w401] -> w28
    shift-left: w30 -> [w403]
    tunnel: [w400] -> _ mode=indexing
    tunnel: w8 -> [w399] mode=indexing
    i -> [w400]
    n125 = call "pb_inst_pbonly.vi"("error in (no error)"=w403, "PB Instruction"=w399, "path in"=w404) -> ("error out"=w401:errorcluster, "path out"=w402:path)  [unwired: 2 in, 5 out]
  }
  n126 = while "Start/Restart Section" {
    stop <- FALSE stop-if-true
    n127 = while {
      tunnel: [errorcluster {"status"=FALSE, "code"=0, "source"=""} ("error in (no error)")] -> w409
      tunnel: [w413] -> w405
      stop <- "start/restart" stop-if-true
      n128 = local read "Path to spinapi.dll"() -> (w413:path)
      n129 = Wait (ms)(milliseconds to wait=u32 10) -> ()  [unwired: 1 out]
    }
    n130 = call "pb_init.vi"("error in (no error)"=w409, "path in"=w405) -> ("error out"=w408:errorcluster, "path out"=w411:path)  [unwired: 1 in, 7 out]
    n131 = call "pb_start.vi"("error in (no error)"=w408, "path in"=w411) -> ("error out"=w407:errorcluster, "path out"=w412:path)  [unwired: 1 in, 7 out]
    n132 = call "pb_close.vi"("error in (no error)"=w407, "path in"=w412) -> ("error out"=w406:errorcluster)  [unwired: 9 out]
    n133 = call <vilib>:"Simple Error Handler.vi"("error in (no error)"=w406) -> ()  [unwired: 1 in, 8 out]
  }
  n134 = while "Stop/Reset Section" {
    stop <- FALSE stop-if-true
    n135 = while {
      tunnel: [errorcluster {"status"=FALSE, "code"=0, "source"=""} ("error in (no error)")] -> w421
      tunnel: [w425] -> w417
      stop <- "stop" stop-if-true
      n136 = local read "Path to spinapi.dll"() -> (w425:path)
      n137 = Wait (ms)(milliseconds to wait=u32 10) -> ()  [unwired: 1 out]
    }
    n138 = call "pb_init.vi"("error in (no error)"=w421, "path in"=w417) -> ("error out"=w420:errorcluster, "path out"=w423:path)  [unwired: 1 in, 7 out]
    n139 = call "pb_stop.vi"("error in (no error)"=w420, "path in"=w423) -> ("error out"=w419:errorcluster, "path out"=w424:path)  [unwired: 8 out]
    n140 = call "pb_close.vi"("error in (no error)"=w419, "path in"=w424) -> ("error out"=w418:errorcluster)  [unwired: 9 out]
    n141 = call <vilib>:"Simple Error Handler.vi"("error in (no error)"=w418) -> ()  [unwired: 1 in, 8 out]
  }
  n142 = call "pb_stop_programming.vi"("error in (no error)"=w28, "path in"=w29) -> ("error out"=w37:errorcluster, "path out"=w38:path)  [unwired: 1 in, 7 out]
  n143 = call "pb_close.vi"("error in (no error)"=w37, "path in"=w38) -> ("error out"=w26:errorcluster)  [unwired: 9 out]
  n144 = call <vilib>:"Simple Error Handler.vi"("error in (no error)"=w26) -> ("error out"=w18:errorcluster)  [unwired: 1 in, 7 out]
  n145 = call-poly <vilib>:"DAQmx Create Virtual Channel.vi"("lines"=tag "Dev1/port0/line1", "error in"=w18) -> ("task out"=w16:refnum<k21>, "error out"=w15:errorcluster)  [unwired: 12 in]
  n146 = call <vilib>:"DAQmx Start Task.vi"("task/channels in"=w16, "error in"=w15) -> ("task out"=w17:refnum<k21>, "error out"=w20:errorcluster)  [unwired: 12 in]
  n147 = while {
    tunnel: w17 -> [w435]
    tunnel: w20 -> [w434]
    shift-right: [w431] -> _
    shift-left: FALSE ("data") -> [w433]
    stop <- FALSE stop-if-true
    n148 = event shown="[1] \"Run\": Value Change" {
      selector: _ -> [_ _]
      dyn-events: _ -> [_ _]
      timeout: 10 -> [_ _]
      event Timeout {
        n149 = event-data() -> ()  [unwired: 1 in, 2 out]
      }
      event "Run": Value Change {
        n150 = event-data() -> ()  [unwired: 1 in, 5 out]
        n151 = local read "Path to spinapi.dll"() -> (w436:path)
        n152 = local read "Run"() -> (w440:bool)
        n153 = call "pb_init.vi"("path in"=w436) -> ("error out"=w441:errorcluster, "path out"=w442:path)  [unwired: 2 in, 7 out]
        n154 = case shown="True" w440 {
          tunnel: w442 -> [w446 w450]
          tunnel: w441 -> [w445 w449]
          tunnel: [w444 w448] -> w438
          tunnel: [w443 w447] -> w437
          frame False {
            n155 = call "pb_stop.vi"("error in (no error)"=w445, "path in"=w446) -> ("error out"=w443:errorcluster, "path out"=w444:path)  [unwired: 8 out]
          }
          frame True {
            n156 = call "pb_start.vi"("error in (no error)"=w449, "path in"=w450) -> ("error out"=w447:errorcluster, "path out"=w448:path)  [unwired: 1 in, 7 out]
          }
        }
        n157 = call "pb_close.vi"("error in (no error)"=w437, "path in"=w438) -> ("error out"=w439:errorcluster)  [unwired: 9 out]
        n158 = call <vilib>:"Simple Error Handler.vi"("error in (no error)"=w439) -> ()  [unwired: 1 in, 8 out]
      }
    }
    n159 = call-poly <vilib>:"DAQmx Read.vi"("task/channels in"=w435, "error in"=w434) -> ("data"=w431:bool)  [unwired: 11 in, 2 out]
    n160 = Not Equal?(x=w431, y=w433) -> (x != y?=w432:bool)
    n161 = case shown="True" w432 {
      tunnel: w431 -> [_ w451]
      frame False {
      }
      frame True {
        n162 = property on="Run" class="Bool (strict)"("Val(Sgnl)"=w451) -> ()  [unwired: 2 in, 2 out]
      }
    }
  }
